vi "GetParam.vi"(8 "error in (no error)":errorcluster caption="entrée d'erreur (pas d'erreur)", 11 "MultiLabelBinarizer.lvclass":refnum<class "MultiLabelBinarizer.lvclass">) -> (0 "error out":errorcluster caption="sortie d'erreur", 2 "MultiLabelBinarizer":T1, 3 "MultiLabelBinarizer.lvclass":refnum<class "MultiLabelBinarizer.lvclass">)   [LabVIEW 2020, in "MultiLabelBinarizer.lvclass"]
doc: "Get Parameters"
uses:
  MultiLabelBinarizer.lvclass
  MultiLabelBinarizer.lvclass/MultiLabelBinarizer.ctl
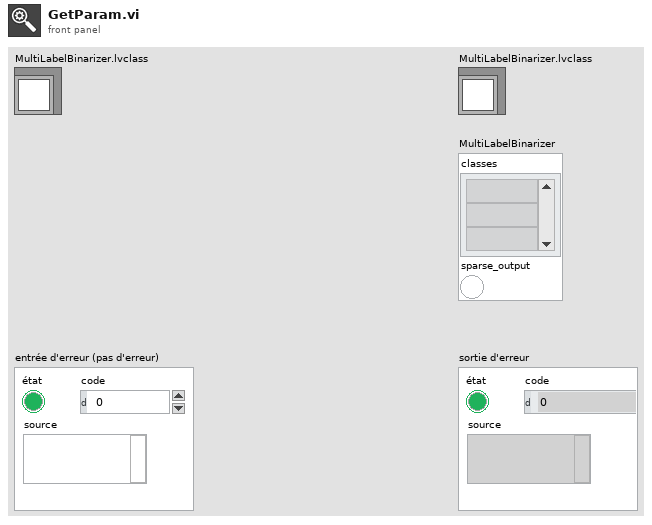
[diagram p1: front panel]
types:
  T1 = cluster{"classes":string[][], "sparse_output":bool}
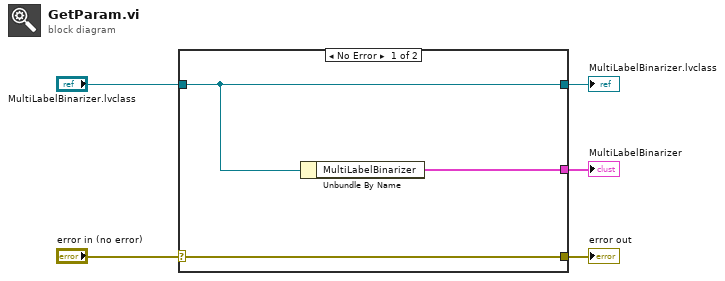
[diagram p0: block diagram]
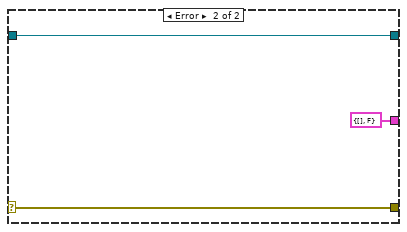
[diagram p2: hidden frame]
diagram:
  n1 = case shown="No Error" "error in (no error)" {
    selector: "error in (no error)" -> [w8 w10]
    tunnel: [w8 w10] -> w4
    tunnel: [w7 w11] -> w2
    tunnel: "MultiLabelBinarizer.lvclass" -> [w7 w11]
    tunnel: [w6 T1 {"classes"=[], "sparse_output"=FALSE} ("MultiLabelBinarizer")] -> w1
    frame No Error {
      n2 = Unbundle By Name(w7) -> ("MultiLabelBinarizer"=w6:T1)
    }
    frame Error {
    }
  }
  "error out" <- w4
  "MultiLabelBinarizer.lvclass" <- w2
  "MultiLabelBinarizer" <- w1
